vi "GetType.vi"(8 "error in (no error)":errorcluster, 11 "Register PVs Msg":refnum<class "Register PVs Msg.lvclass">) -> (0 "error out":errorcluster, 2 "Data Sample":variant, 3 "Register PVs Msg":refnum<class "Register PVs Msg.lvclass">)   [LabVIEW 2015, in "CS++PVProxy.lvlib" / "Register PVs Msg.lvclass"]
uses:
  Register PVs Msg.lvclass
  Register PVs Msg.lvclass/Register PVs Msg.ctl
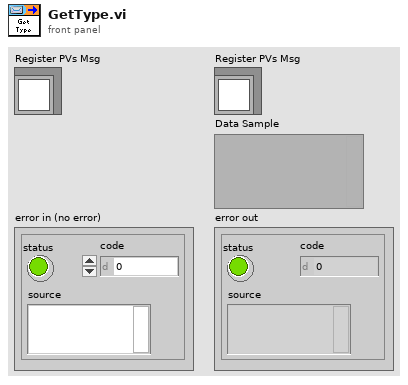
[diagram p1: front panel]
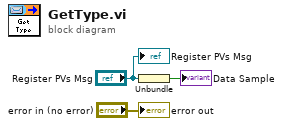
[diagram p0: block diagram]
diagram:
  n1 = Unbundle("Register PVs Msg") -> (→"Data Sample":bool)
  "error out" <- "error in (no error)"
  "Register PVs Msg" <- "Register PVs Msg"
